vi "Initialize Dependencies Attribute.vi"() -> (3 "Attribute.Dependencies":refnum<class "Attribute.Dependencies.lvclass">)   [LabVIEW 2013, in "SMOAttributes.lvlib" / "Attribute.Dependencies.lvclass"]
uses:
  Attribute.Dependencies.lvclass
  Definitions/def.SMO/Scope -- Enum.ctl
  Attribute/Attribute.lvclass/Attribute.ctl
  Attribute.Dependencies.lvclass/Attribute.Dependencies.ctl
  Attribute/Attribute.lvclass
  Definitions/def.SMO/def.SMO.lvclass
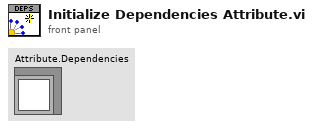
[diagram p1: front panel]
types:
  T1 = typedef "def.SMO.lvclass/Scope -- Enum.ctl" = enum16{"Public", "Protected", "Private"}
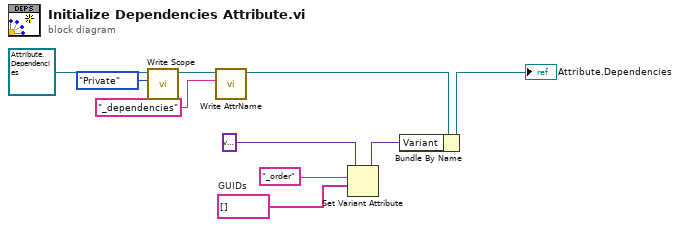
[diagram p0: block diagram]
diagram:
  w1 = string[] []  # GUIDs
  n1 = call "Write Scope.vi"("Scope"=Scope_--_Enum."Private", "Attribute in"=refnum<class "Attribute.Dependencies.lvclass"> refnum ("Attribute.Owner in")) -> ("Attribute out"=w9:refnum<class "Attribute.Dependencies.lvclass">)  [unwired: 9 in]
  n2 = call "Write AttrName.vi"("Attribute Name"="_dependencies", "Attribute in"=w9) -> ("Attribute out"=w7:refnum<class "Attribute.Dependencies.lvclass">)  [unwired: 9 in]
  n3 = Set Variant Attribute(Variant=variant, name="_order" ("Attribute Name"), value=w1) -> (Variant out=w3:variant)  [unwired: 1 in, 2 out]
  n4 = Bundle By Name(cluster=w7, "Variant"=w3) -> (→"Attribute.Dependencies":refnum<class "Attribute.Dependencies.lvclass">)
